vi "TESTJOG.vi"() -> ()   [LabVIEW 2016]
uses:
  <vilib>/regexp/Match Regular Expression.xnode
  <vilib>/vision/driver/NI_Vision_Acquisition_Software.lvlib
panel:
  out "error out":errorcluster
  in  "error in (no error)":errorcluster
  in  "Confirm Position":bool
  in  "Right":bool
  in  "Backward":bool
  in  "Forward":bool
  in  "Left":bool
  out "Image Out":T1(plugin-control)
  in  "Camera Name":refnum<k21>="cam0" caption="IMAQdx Session"
  in  "Jog step size":T2={"X [mm]"=0.001, "Y [mm]"=0.001, "Z [mm]"=0.001}
  in  "stop":bool
  out "Moving":bool
  out "Stave origin":T2
  out "Current stage position [mm]":cluster{"X":dbl, "Y":dbl, "Z":dbl}
  in  "Axis Speeds":T3={"X [mm/s]"=10.0, "Y [mm/s]"=10.0, "Z [mm/s]"=10.0}
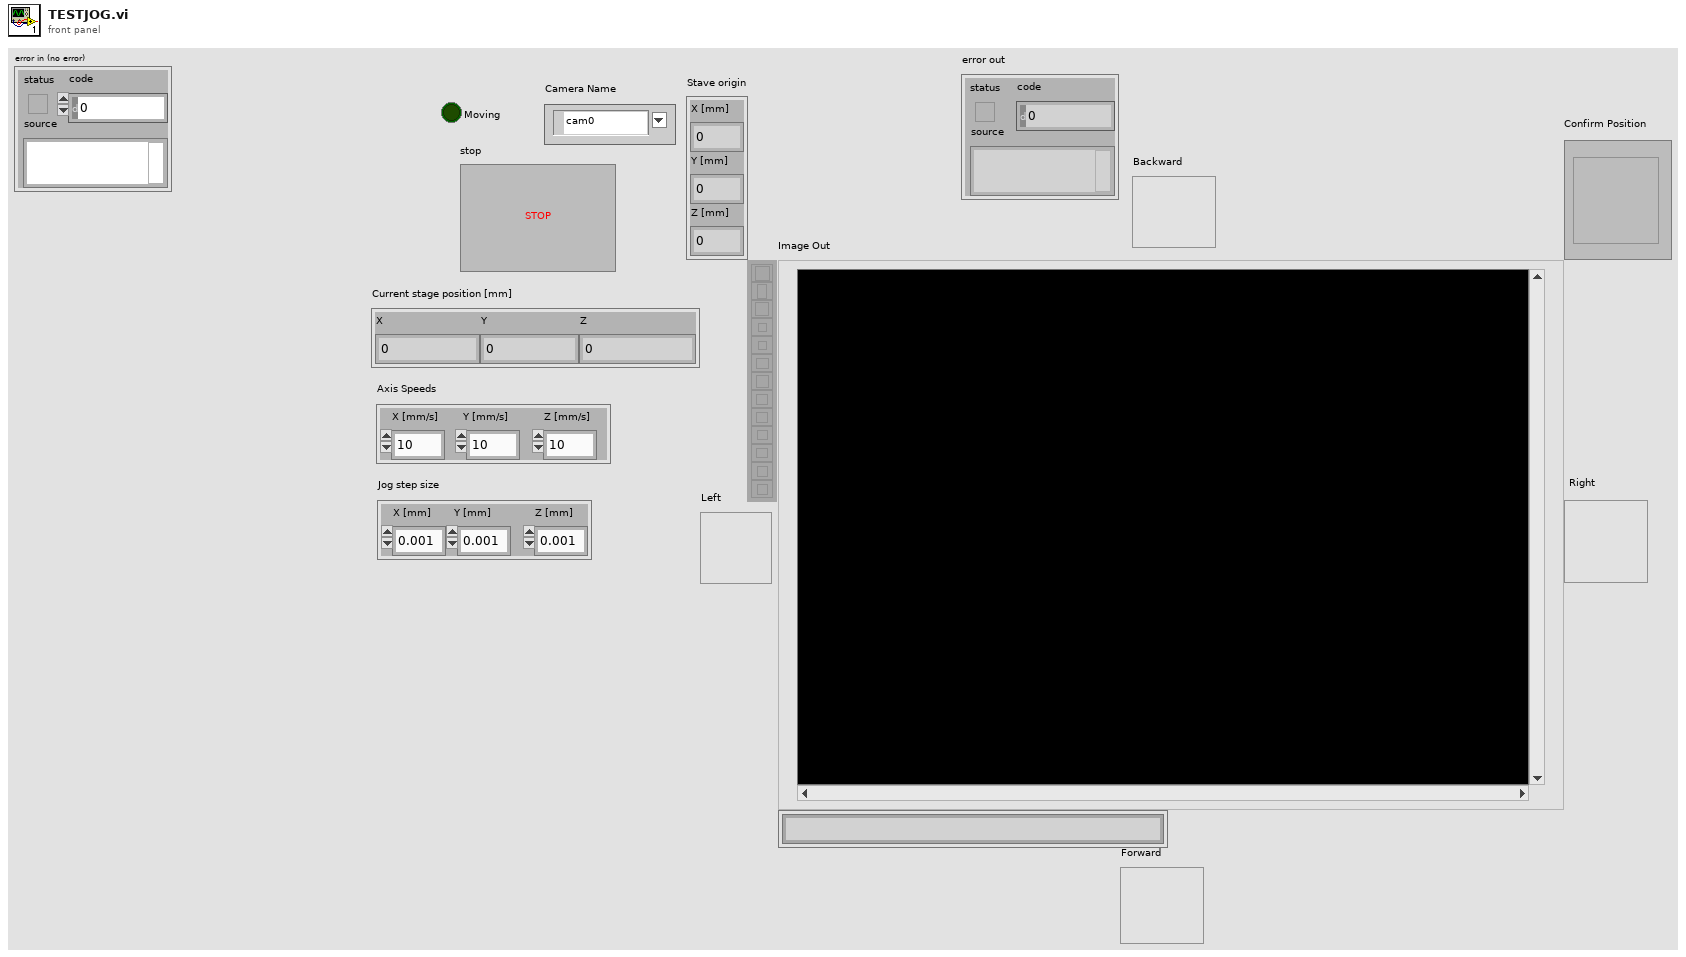
[diagram p1: front panel]
types:
  T1 = typedef "IMAQ Image.ctl" = refnum<image>
  T2 = cluster{"X [mm]":dbl, "Y [mm]":dbl, "Z [mm]":dbl}
  T3 = cluster{"X [mm/s]":dbl, "Y [mm/s]":dbl, "Z [mm/s]":dbl}
  T4 = typedef "IMAQdx.ctl" = refnum<k21>
  T5 = cluster{"Final X":dbl, "Final Y":dbl, "Final Z":dbl}
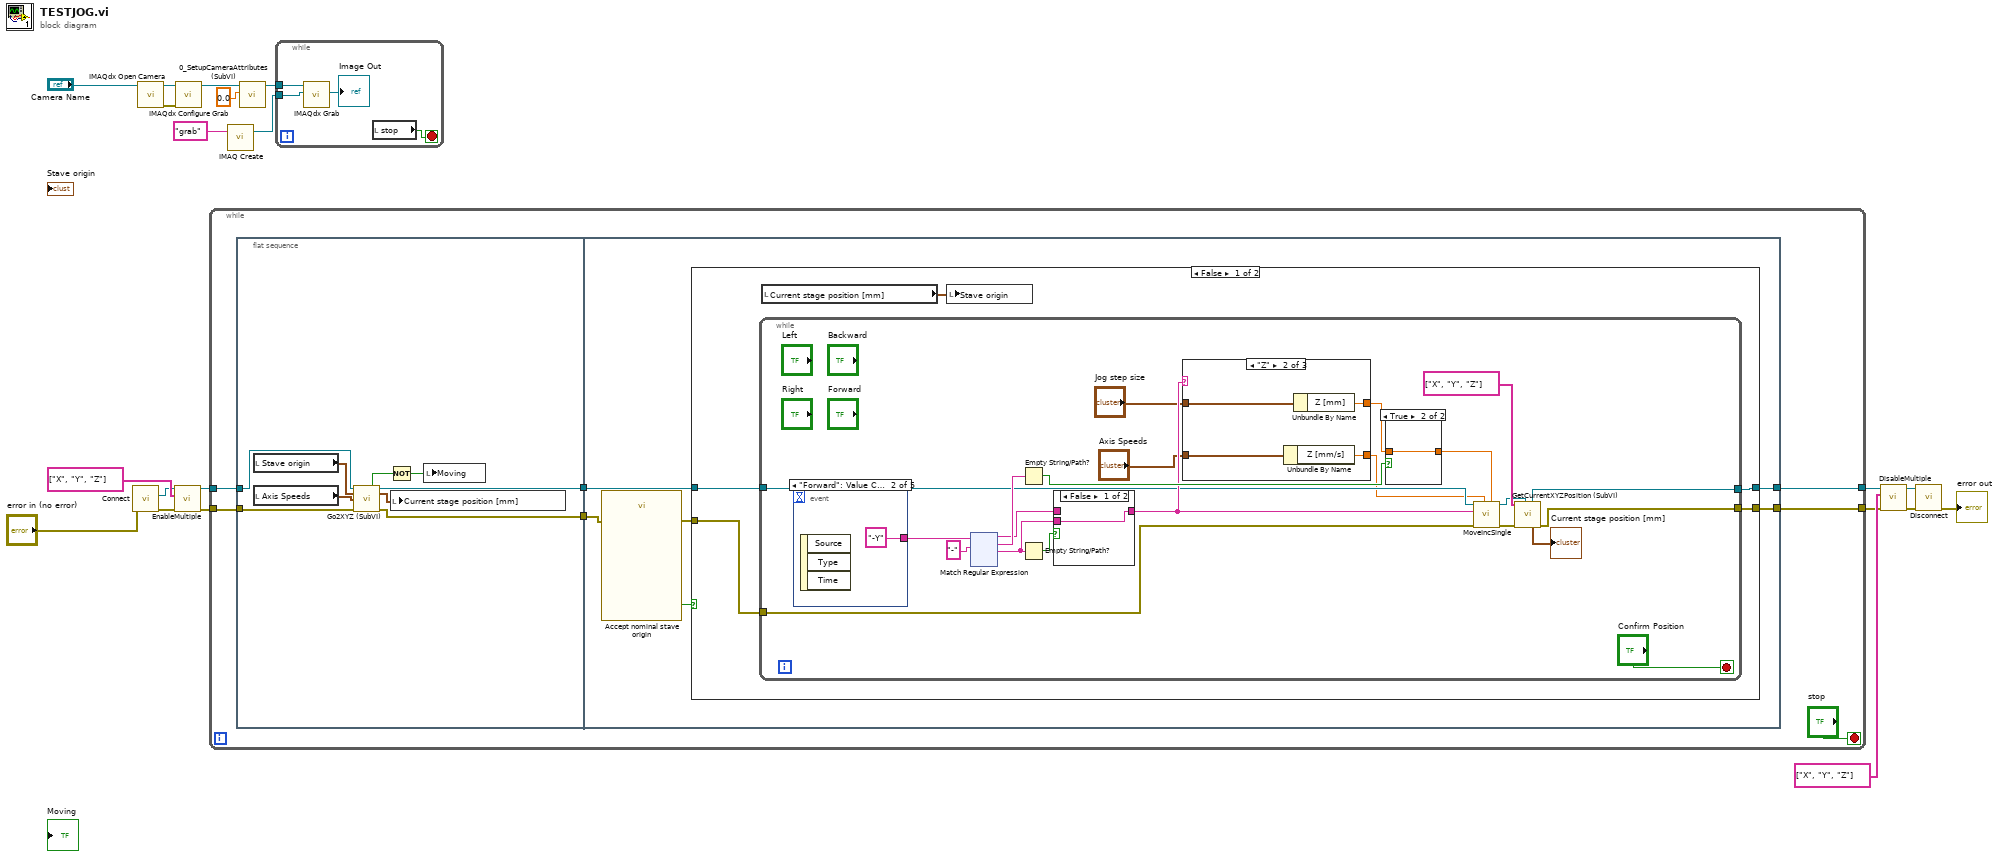
[diagram p0: block diagram]
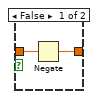
[diagram p3: hidden frame]
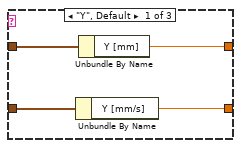
[diagram p4: hidden frame]
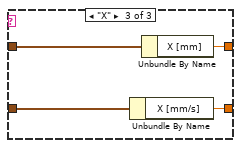
[diagram p5: hidden frame]
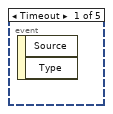
[diagram p6: hidden frame]
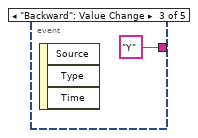
[diagram p7: hidden frame]
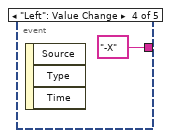
[diagram p8: hidden frame]
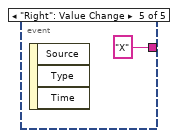
[diagram p9: hidden frame]
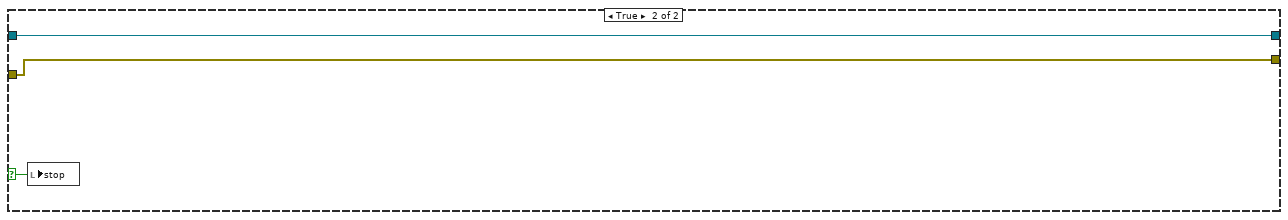
[diagram p10: hidden frame]
diagram:
  n1 = call "Connect.vi"("error in (no error)"="error in (no error)") -> ("error out"=w9:errorcluster, "controller"=w11:refnum<k24>)  [unwired: 9 in]
  n2 = call <vilib>:"IMAQdx Open Camera.vi"("Session In"="Camera Name") -> ("error out"=w19:errorcluster, "Session Out"=w20:T4)  [unwired: 2 in, 7 out]
  n3 = call "EnableMultiple.vi"("error in (no error)"=w9, "axis names"=string[] ["X", "Y", "Z"], "controller in"=w11) -> ("error out"=w8:errorcluster, "controller out"=w10:refnum<k24>)  [unwired: 7 in]
  n4 = call <vilib>:"IMAQdx Configure Grab.vi"("error in"=w19, "Session In"=w20) -> ("Session Out"=w15:T4)  [unwired: 9 out]
  n5 = while {
    tunnel: w10 -> [w26]
    tunnel: w8 -> [w24]
    tunnel: [w23] -> w4
    tunnel: [w21] -> w2
    stop <- "stop" stop-if-true
    n6 = flat-sequence {
      tunnel: w26 -> [w31]
      tunnel: [w30] -> w25
      tunnel: w24 -> [w29]
      tunnel: [w28] -> w22
      tunnel: w25 -> [w41]
      tunnel: [w40] -> w23
      tunnel: w22 -> [w39]
      tunnel: [w37] -> w21
      frame #0 {
        n7 = local read "Stave origin"() -> (w33:T2)
        n8 = local read "Axis Speeds"() -> (w32:T3)
        n9 = call "Go2XYZ (SubVI).vi"(".NET Refnum in"=w31, "Go to Coordinates"=w33, "Axis Speeds"=w32, "error in (no error)"=w29) -> ("completed"=w35:bool, ".NET Refnum out"=w30:refnum<k24>, "Final Position"=w34:T5, "error out"=w28:errorcluster)  [unwired: 7 in, 1 out]
        n10 = Not(x=w35) -> (.not. x?=w36:bool)
        n11 = local write "Current stage position [mm]"(w34) -> ()
        n12 = local write "Moving"(w36) -> ()
      }
      frame #1 {
        n13 = call "Accept nominal stave origin"("error in (no error)"=w39) -> ("Accept stave origin"=w42:bool, "error out"=w38:errorcluster)  [unwired: 16 in, 1 out]
        n14 = case shown="False" w42 {
          selector: w42 -> [_ w207]
          tunnel: w41 -> [w46 w206]
          tunnel: [w45 w206] -> w40
          tunnel: w38 -> [w44 w205]
          tunnel: [w43 w205] -> w37
          frame False {
            n15 = while {
              tunnel: w46 -> [w55]
              tunnel: [w67] -> w45
              tunnel: w44 -> [w49]
              tunnel: [w48] -> w43
              stop <- "Confirm Position" stop-if-true
              n16 = event shown="[1] \"Forward\": Value Change" {
                selector: _ -> [_ _ _ _ _]
                dyn-events: _ -> [_ _ _ _ _]
                timeout: _ -> [_ _ _ _ _]
                tunnel: [_ "-Y" "Y" "-X" "X"] -> w56
                event Timeout {
                  n17 = event-data() -> ()  [unwired: 1 in, 2 out]
                }
                event "Forward": Value Change {
                  n18 = event-data() -> ()  [unwired: 1 in, 3 out]
                }
                event "Backward": Value Change {
                  n19 = event-data() -> ()  [unwired: 1 in, 3 out]
                }
                event "Left": Value Change {
                  n20 = event-data() -> ()  [unwired: 1 in, 3 out]
                }
                event "Right": Value Change {
                  n21 = event-data() -> ()  [unwired: 1 in, 3 out]
                }
              }
              n22 = xnode "Match Regular Expression"("input string"=w56, "regular expression"="-") -> ("before match"=w57:string, "whole match"=w62:string, "after match"=w58:string)  [unwired: 4 in, 2 out]
              n23 = Empty String/Path?(string/path=w62) -> (empty?=w61:bool)
              n24 = Empty String/Path?(string/path=w58) -> (empty?=w60:bool)
              n25 = case shown="False" w60 {
                tunnel: w57 -> [_ w71]
                tunnel: [w70 w71] -> w59
                tunnel: w58 -> [w70 _]
                frame False {
                }
                frame True {
                }
              }
              n26 = case shown="\"Z\"" w59 {
                tunnel: [w191 w195 w200] -> w65
                tunnel: [w192 w196 w199] -> w50
                tunnel: "Jog step size" -> [w190 w194 w198]
                tunnel: "Axis Speeds" -> [w189 w193 w197]
                frame "Y", Default {
                  n27 = Unbundle By Name(w189) -> ("Y [mm/s]"=w192:dbl)
                  n28 = Unbundle By Name(w190) -> ("Y [mm]"=w191:dbl)
                }
                frame "Z" {
                  n29 = Unbundle By Name(w193) -> ("Z [mm/s]"=w196:dbl)
                  n30 = Unbundle By Name(w194) -> ("Z [mm]"=w195:dbl)
                }
                frame "X" {
                  n31 = Unbundle By Name(w197) -> ("X [mm/s]"=w199:dbl)
                  n32 = Unbundle By Name(w198) -> ("X [mm]"=w200:dbl)
                }
              }
              n33 = case shown="True" w61 {
                tunnel: w65 -> [w186 w188]
                tunnel: [w187 w188] -> w64
                frame False {
                  n34 = Negate(x=w186) -> (-x=w187:dbl)
                }
                frame True {
                }
              }
              n35 = call "MoveIncSingle.vi"("distance"=w64, "speed"=w50, "error in (no error)"=w49, "axis name"=w59, "controller in"=w55) -> ("error out"=w53:errorcluster, "controller out"=w54:refnum<k24>)  [unwired: 5 in]
              n36 = call "GetCurrentXYZPosition (SubVI).vi"(".NET Refnum in - Device"=w54, "error in (no error)"=w53, "Axes Names"=string[] ["X", "Y", "Z"]) -> ("error out"=w48:errorcluster, "Current stage position"=→"Current stage position [mm]":T2, ".NET Refnum out  - Device"=w67:refnum<k24>)  [unwired: 3 in, 3 out]
            }
            n37 = local read "Current stage position [mm]"() -> (w47:cluster{"X":dbl, "Y":dbl, "Z":dbl})
            n38 = local write "Stave origin"(w47) -> ()
          }
          frame True {
            n39 = local write "stop"(w207) -> ()
          }
        }
      }
    }
  }
  n40 = call "IMAQ Create"("Image Name"="grab") -> ("New Image"=w14:T1)  [unwired: 4 in, 1 out]
  n41 = call "0_SetupCameraAttributes (SubVI).vi"("Gain"=0.0, "Camera session in"=w15) -> ("Camera session out"=w13:T4)  [unwired: 8 in, 1 out]
  n42 = while {
    tunnel: w14 -> [w210]
    tunnel: w13 -> [w209]
    stop <- w211 stop-if-true
    n43 = call <vilib>:"IMAQdx Grab.vi"("Image In"=w210, "Session In"=w209) -> ("Image Out"=→"Image Out":T1)  [unwired: 2 in, 7 out]
    n44 = local read "stop"() -> (w211:bool)
  }
  n45 = call "DisableMultiple.vi"("error in (no error)"=w2, "axis names"=string[] ["X", "Y", "Z"], "controller in"=w4) -> ("error out"=w7:errorcluster, "controller out"=w6:refnum<k24>)  [unwired: 7 in]
  n46 = call "Disconnect.vi"("error in (no error)"=w7, "controller"=w6) -> ("error out"=→"error out":errorcluster)  [unwired: 9 in]
